vi "COMLOGQueue-Dequeue.vi"(5 "COM(Constant)":string, 6 "Error in":errorcluster caption="Error in (no error)", 7 "timeout in ms (-1)":i32=500) -> (0 "Error out":errorcluster, 1 "timed out?":bool, 2 "element":string)   [LabVIEW 2020]
uses:
  8d7bb56f-8634-4bdc-b000-1a4d4596e07b.vi
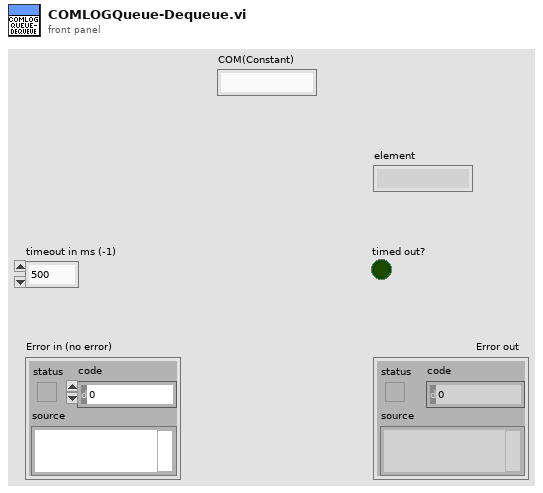
[diagram p1: front panel]
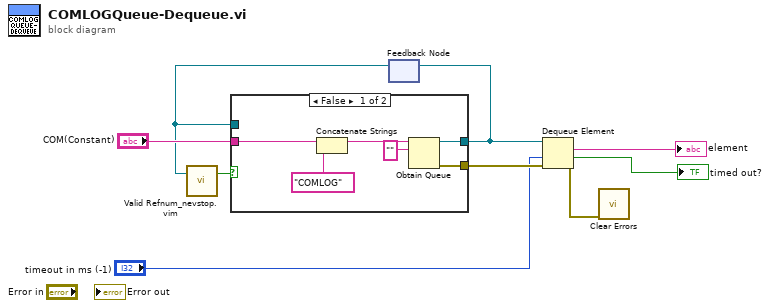
[diagram p0: block diagram]
diagram:
  n1 = feedback #1() -> (w7:refnum<queue>)  [unwired: 1 in]
  n2 = call "Valid Refnum_nevstop.vim"("number/path/refnum"=w7) -> ("Valid Number/Path/Refnum"=w8:bool)  [unwired: 2 in]
  n3 = case shown="False" w8 {
    tunnel: "COM(Constant)" -> [w15 _]
    tunnel: [w13 w16] -> w6
    tunnel: w7 -> [_ w16]
    tunnel: [w10 _] -> w5
    frame False {
      n4 = Concatenate Strings(w15, "COMLOG" ("string")) -> (w12:string)
      n5 = Obtain Queue(name (unnamed)=w12, element data type="") -> (queue out=w13:refnum<queue>, error out=w10:errorcluster)  [unwired: 3 in, 1 out]
    }
    frame True {
    }
  }
  n6 = feedback-in #1(w6) -> ()
  n7 = Dequeue Element(queue=w6, timeout in ms (-1)="timeout in ms (-1)", error in (no error)=w5) -> (element=→"element":string, timed out?=→"timed out?":bool, error out=w3:errorcluster)  [unwired: 1 out]
  n8 = call <vilib>:"Clear Errors.vi"("error in (no error)"=w3) -> ()  [unwired: 5 in, 2 out]
